vi "Add controls and indicators.vi"() -> ()   [LabVIEW 2020]
uses:
  <vilib>/Utility/traverseref.llb/TRef TravTarget.ctl
  <vilib>/Utility/config.llb/Read Key (String).vi
  <vilib>/Utility/config.llb/NI_LVConfig.lvlib
  <vilib>/Utility/traverseref.llb/VI Scripting - Traverse.lvlib
panel:
  out "section exists?":bool
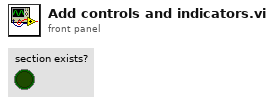
[diagram p1: front panel]
types:
  T1 = typedef "NI_LVConfig.lvlib/Config Data RefNum.ctl" = refnum<k1>
  T2 = typedef "TRef TravTarget.ctl" = enum16{"FP", "BD", "Other"}
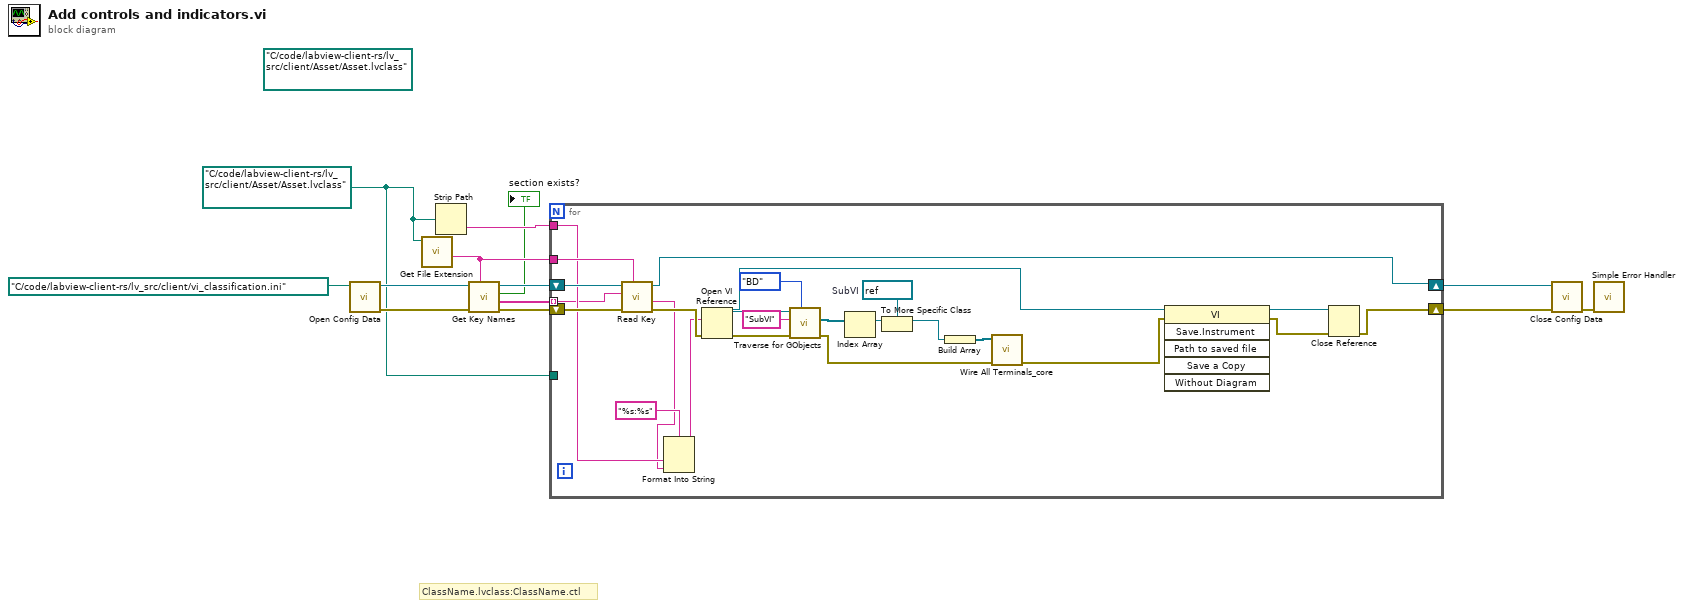
[diagram p0: block diagram]
diagram:
  (unwired) path "C:/code/labview-client-rs/lv_src/client/Asset/Asset.lvclass" ("Path")
  w1 = path "C:/code/labview-client-rs/lv_src/client/Asset/Asset.lvclass" ("Path")
  # "ClassName.lvclass:ClassName.ctl"
  n1 = call <vilib>:"Open Config Data.vi"("configuration file path"=path "C:/code/labview-client-rs/lv_src/client/vi_classification.ini") -> ("error out"=w11:errorcluster, "refnum"=w2:T1)  [unwired: 8 in, 1 out]
  n2 = call <vilib>:"Get File Extension.vi"("file"=w1) -> ("filename without extension"=w8:string)  [unwired: 6 in, 4 out]
  n3 = Strip Path(path=w1) -> (name=w6:string)  [unwired: 1 out]
  n4 = call <vilib>:"Get Key Names.vi"("section"=w8, "error in (no error)"=w11, "refnum"=w2) -> ("error out"=w7:errorcluster, "key names"=w10:string[], "section exists?"=→"section exists?":bool, "refnum out"=w9:T1)  [unwired: 5 in]
  n5 = for {
    tunnel: w10 -> [w27] mode=indexing
    tunnel: w8 -> [w35]
    tunnel: w6 -> [w28]
    shift-right: [w33] -> w5
    shift-left: w9 -> [w34]
    shift-right: [w31] -> w4
    shift-left: w7 -> [w32]
    tunnel: w1 -> [_]
    w20 = refnum<vi> refnum  # SubVI
    n6 = call-poly <vilib>:"Read Key.vi"("section"=w35, "error in (no error)"=w32, "key"=w27, "refnum"=w34) -> ("error out"=w30:errorcluster, "value"=w25:string, "refnum out"=w33:T1)  [unwired: 4 in, 1 out]
    n7 = Format Into String(format string="%s:%s", w28, w25) -> (resulting string=w26:string)  [unwired: 2 in, 1 out]
    n8 = Open VI Reference(vi path=w26, error in (no error)=w30) -> (vi reference=w15:refnum<vi>, error out=w24:errorcluster)  [unwired: 4 in]
    n9 = call <vilib>:"Traverse for GObjects.vi"("Traverse Target"=TRef_TravTarget."BD", "error in (no error)"=w24, "Class Name"="SubVI", "VI Refnum"=w15) -> ("error out"=w17:errorcluster, "References"=w22:refnum<vi>[])  [unwired: 4 in, 2 out]
    n10 = Index Array(array=w22) -> (element=w21:refnum<vi>)  [unwired: 1 in]
    n11 = To More Specific Class(target class=w20, reference=w21) -> (specific class reference=w19:refnum<vi>)  [unwired: 1 in, 1 out]
    n12 = Build Array(w19) -> (w18:refnum<vi>[])
    n13 = call <vilib>:"Wire All Terminals_core.vi"("error in (no error)"=w17, "SelList[]"=w18) -> ("error out"=w16:errorcluster)  [unwired: 8 in, 1 out]
    n14 = invoke class="VI" method="Save.Instrument"(reference=w15, error in=w16) -> (reference out=w36:refnum<vi>, error out=w37:errorcluster)  [unwired: 4 in, 4 out]
    n15 = Close Reference(reference=w36, error in (no error)=w37) -> (error out=w31:errorcluster)
  }
  n16 = call <vilib>:"Close Config Data.vi"("error in (no error)"=w4, "refnum"=w5) -> ("error out"=w13:errorcluster)  [unwired: 8 in, 1 out]
  n17 = call <vilib>:"Simple Error Handler.vi"("error in (no error)"=w13) -> ()  [unwired: 4 in, 5 out]
